vi "Boolean Functions.vi"() -> ()   [LabVIEW 2019]
doc: "This example shows how the And function operates with different data types. These concepts also apply to the Or, Exclusive Or, Not, Not And, Not Or, Not Exclusive Or, and Implies functions."
uses:
  <vilib>/silver_ctls/ArrayMatrixCluster/Real Matrix NI_Silver.ctl
panel:
  in  "Tab Control":T1(tab)
  out "X and Y?":bool
  in  "Boolean Y":bool=TRUE
  in  "Boolean X":bool=TRUE
  out "X and Y? (array)":bool[](array[boolean])
  in  "Input Array Y":bool[](array[boolean])=[FALSE, FALSE, TRUE, TRUE]
  in  "Input Array X":bool[](array[boolean])=[FALSE, TRUE, FALSE, TRUE]
  out "X and Y? (cluster)":T2
  in  "Input Cluster Y":T2={"Boolean 1"=TRUE, "Boolean 2"=TRUE, "Boolean 3"=FALSE, "Boolean 4"=FALSE}
  in  "Input Cluster X":T2={"Boolean 1"=TRUE, "Boolean 2"=FALSE, "Boolean 3"=TRUE, "Boolean 4"=FALSE}
  out "Result Binary":u32 format="%08b"
  out "Input Binary":u32 format="%08b"
  out "Mask Binary":u32 format="%08b"
  in  "Input":u32=46
  in  "Mask":u32=26
  out "Result":u32
  in  "Array Y":u32[](array[numeric])=[2, 2, 2, 2] format="%02b"
  in  "Array X":u32[](array[numeric])=[2, 1, 3, 0] format="%02b"
  out "Array of X and Y":u32[](array[numeric]) format="%02b"
  out "Matrix X and Y":i32[][](array[numeric])
  in  "Matrix Y":T3=[[26.0, 46.0], [5.0, 7.0]]
  in  "Matrix X":T3=[[46.0, 26.0], [1.0, 2.0]]
  # "Overview: Demonstrates how the And function operates with different data types.\nInstructions:\n1. Run the VI.\n2. Examine the different cases.\n3. Although this example demonstrates the And function, the concepts also apply to other Boolean functions including the Compound Arithmetic function which can do Boolean operations on more than two inputs."
  # "The most common use of the And function is with two Booleans. The result is true only if both of the inputs are true."
  # "When comparing arrays, the And function compares each element to its corresponding value in the second array."
  # "When comparing clusters, the And function compares each element to its corresponding value in the second cluster."
  # "The And function acts as a masking function when you use it with two numerics."
  # "When comparing arrays of numerics, the And function masks each element in X with the corresponding value in the second array."
  # "The And function used on a matrix of numerics acts just like it does in individual numerics.  It masks each number by its corresponding input in the second matrix. Arrays will act the exact same way."
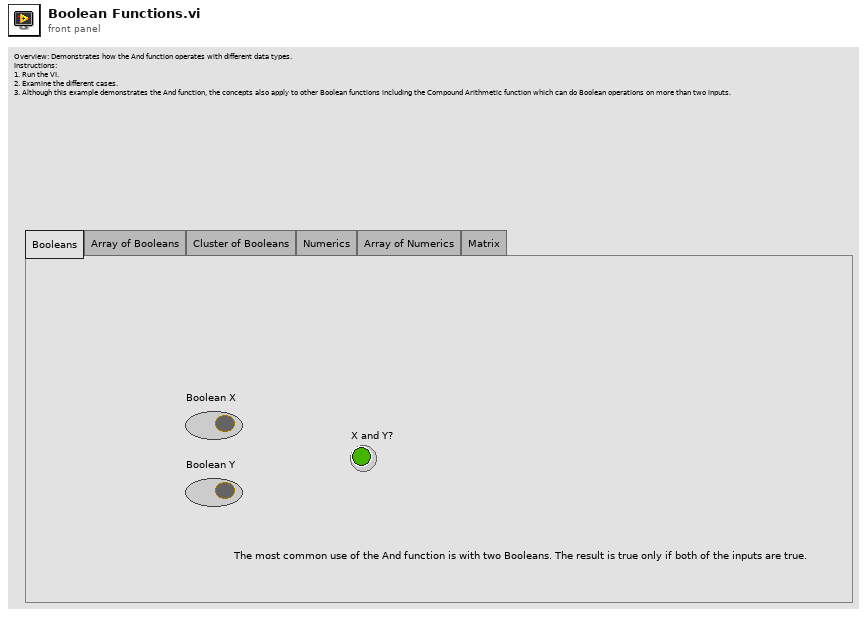
[diagram p1: front panel]
types:
  T1 = enum32{"Booleans", "Array of Booleans", "Cluster of Booleans", "Numerics", "Array of Numerics", "Matrix"}
  T2 = cluster{"Boolean 1":bool, "Boolean 2":bool, "Boolean 3":bool, "Boolean 4":bool}
  T3 = typedef "Real Matrix NI_Silver.ctl" = dbl[][]
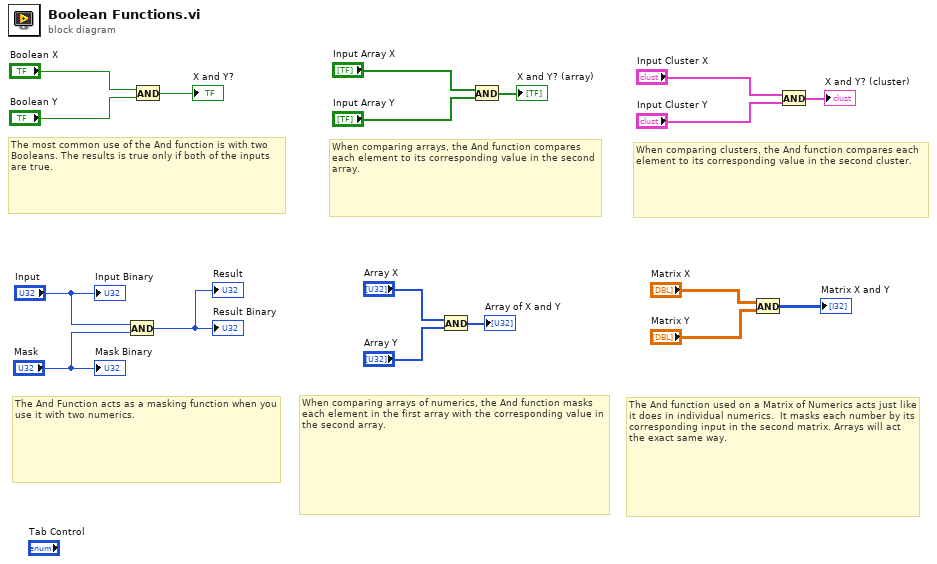
[diagram p0: block diagram]
diagram:
  # "When comparing arrays, the And function compares each element to its corresponding value in the second array."
  # "When comparing clusters, the And function compares each element to its corresponding value in the second cluster."
  # "When comparing arrays of numerics, the And function masks each element in the first array with the corresponding value in the second array."
  # "The And function used on a Matrix of Numerics acts just like it does in individual numerics.  It masks each number by its corresponding input in the second matrix. Arrays will act the exact same way."
  # "The And Function acts as a masking function when you use it with two numerics."
  # "The most common use of the And function is with two Booleans. The results is true only if both of the inputs are true."
  n1 = And(x="Input", y="Mask") -> (x .and. y?=→"Result" →"Result Binary":u32)
  n2 = And(x="Boolean X", y="Boolean Y") -> (x .and. y?=→"X and Y?":bool)
  n3 = And(x="Array X", y="Array Y") -> (x .and. y?=→"Array of X and Y":u32[])
  n4 = And(x="Input Array X", y="Input Array Y") -> (x .and. y?=→"X and Y? (array)":bool[])
  n5 = And(x="Matrix X", y="Matrix Y") -> (x .and. y?=→"Matrix X and Y":i32[][])
  n6 = And(x="Input Cluster X", y="Input Cluster Y") -> (x .and. y?=→"X and Y? (cluster)":T2)
  "Mask Binary" <- "Mask"
  "Input Binary" <- "Input"
